vi "Transfer Image Metadata To Host.vi"(0 "image metadata":T1, 1 "reset":bool, 2 "image metadata dma fifo":refnum<k21>, 9 "input valid":bool) -> (4 "overflow":bool, 14 "ready for input":bool)   [LabVIEW 2020, in "GettingStarted_Common_148X_FPGA.lvlib"]
uses:
  GettingStarted_Common_148X_FPGA.lvlib
  Types/Image Metadata.ctl
  <instrlib>/FlexRIO/CSI-2/v2/Common/Types/LLP Data Type.ctl
  <vilib>/rvi/DataTransferAndStorage/Container/Common/niFpgaContainerExecOnDevCompGetState.vi
  <vilib>/rvi/Emulation/niFpgaSctlEmulationGetInTimedLoop.vi
  <vilib>/rvi/errors/niFpgaSetErrorForExecOnDevCompSimple.vi
  <vilib>/rvi/eio/common/nirviEmuReportErrorAndStop.vi
  <vilib>/rvi/interface/RandomDataEmulation/nirviRandomDataAcquireLock.vi
  <vilib>/rvi/interface/RandomDataEmulation/nirviRandomDataQueueStore.vi
  <vilib>/rvi/interface/RandomDataEmulation/nirviRandomDataReleaseLock.vi
  <vilib>/rvi/interface/RandomDataEmulation/nirviFPGAContextMergeError.vi
  <vilib>/rvi/interface/RandomDataEmulation/nirviRandomDataCheckExitLoopConditions.vi
  <vilib>/express/rvi/timingcommon/nirviCommon.vi
  <vilib>/rvi/interface/RandomDataEmulation/niFpgaRandomDataHandleErrors.vi
  <vilib>/rvi/DataTransferAndStorage/Container/XNode/niFpgaContainer.xnode
  <vilib>/rvi/FIFO/Fifo_Resource/niFpgaFifoEmulationRefInMultiElement.vi
  <instrlib>/_niInstr/Basic Elements/v1/FPGA/niInstr Basic Elements v1 FPGA.lvlib
  <instrlib>/FlexRIO/CSI-2/v2/Common/NI CSI-2 API Common v2.lvlib
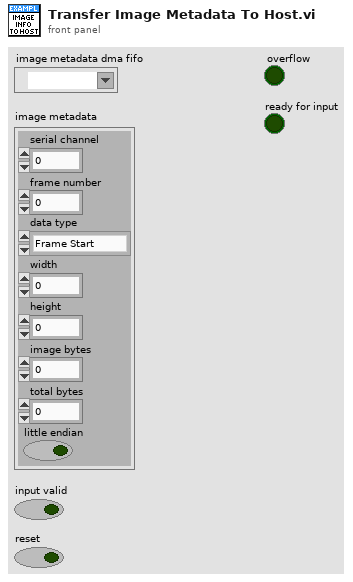
[diagram p1: front panel]
types:
  T1 = typedef "GettingStarted_Common_148X_FPGA.lvlib/Image Metadata.ctl" = cluster{"serial channel":fxp<+,3,3>, "frame number":u16, "data type":T2, "width":u16, "height":u16, "image bytes":u32, "total bytes":u32, "little endian":bool}
  T2 = typedef "NI CSI-2 API Common v2.lvlib/LLP Data Type.ctl" = enum8{"Frame Start", "Frame End", "Line Start", "Line End", "End of Transmission", "Reserved 0", "Reserved 1", "Reserved 2", "Generic Short Packet 1", "Generic Short Packet 2", "Generic Short Packet 3", "Generic Short Packet 4", "Generic Short Packet 5", "Generic Short Packet 6", "Generic Short Packet 7", "Generic Short Packet 8", "Null", "Blanking Data", "Embedded 8-bit non Image Data", "Generic Long Packet 1", "Generic Long Packet 2", "Generic Long Packet 3", "Generic Long Packet 4", "Reserved 3", "YUV420 8-bit", "YUV420 10-bit", "Legacy YUV420 8-bit", "Reserved 4", "YUV420 8-bit Chroma Shifted", "YUV420 10-bit Chroma Shifted", "YUV422 8-bit", "YUV422 10-bit", "RGB444", "RGB555", "RGB565", "RGB666", "RGB888", "Reserved 5", "Reserved 6", "RAW 24", "RAW 6", "RAW 7", "RAW 8", "RAW 10", "RAW 12", "RAW 14", "RAW 16", "RAW 20", "User Defined 8-bit Data 1", "User Defined 8-bit Data 2", "User Defined 8-bit Data 3", "User Defined 8-bit Data 4", "User Defined 8-bit Data 5", "User Defined 8-bit Data 6", "User Defined 8-bit Data 7", "User Defined 8-bit Data 8", "USL Command", "Reserved 7", "Reserved 8", "Reserved 9", "Reserved 10", "Reserved 11", "Reserved 12", "LRTE EPD Spacer"}
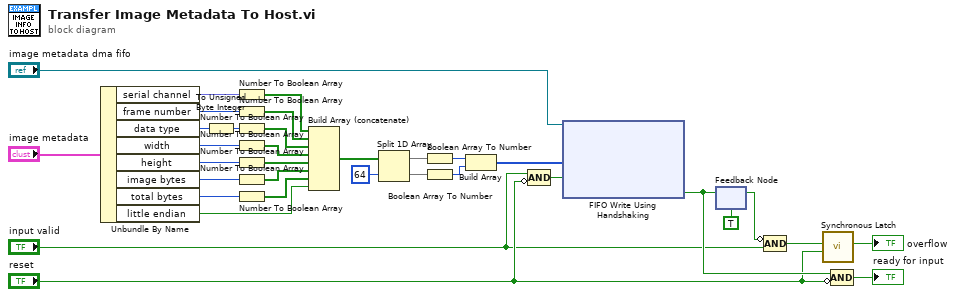
[diagram p0: block diagram]
diagram:
  n1 = Unbundle By Name("image metadata") -> ("serial channel"=w2:fxp<+,3,3>, "frame number"=w32:u16, "data type"=w31:T2, "width"=w30:u16, "height"=w29:u16, "image bytes"=w28:u32, "total bytes"=w21:u32, "little endian"=w4:bool)
  n2 = To Unsigned Byte Integer(number=w31) -> (unsigned 8bit integer=w27:u8)
  n3 = Number To Boolean Array(number=w2) -> (Boolean array=w1:bool[])
  n4 = Number To Boolean Array(number=w32) -> (Boolean array=w26:bool[])
  n5 = Number To Boolean Array(number=w27) -> (Boolean array=w25:bool[])
  n6 = Number To Boolean Array(number=w30) -> (Boolean array=w24:bool[])
  n7 = Number To Boolean Array(number=w29) -> (Boolean array=w23:bool[])
  n8 = Number To Boolean Array(number=w28) -> (Boolean array=w22:bool[])
  n9 = Number To Boolean Array(number=w21) -> (Boolean array=w3:bool[])
  n10 = Build Array (concatenate)(w1, w26, w25, w24, w23, w22, w3, w4) -> (w20:bool[])
  n11 = Split 1D Array(array=w20, index=64) -> (first subarray=w18:bool[], second subarray=w17:bool[])
  n12 = Boolean Array To Number(Boolean array=w18) -> (number=w16:u64)
  n13 = Boolean Array To Number(Boolean array=w17) -> (number=w15:u64)
  n14 = Build Array(w16, w15) -> (w14:u64[])
  n15 = Compound Arithmetic op=AND("input valid", invert "reset") -> (w5:bool)
  n16 = xnode ("FIFO Write Using Handshaking")("Element"=w14, "Input Valid"=w5, "FIFO In"="image metadata dma fifo") -> ("Ready for Input"=w10:bool)  [unwired: 1 out]
  n17 = feedback-in #1(w10) -> ()
  n18 = feedback #1(TRUE ("Ready for Input")) -> (w9:bool)
  n19 = Compound Arithmetic op=AND(invert w9, "input valid") -> (w12:bool)
  n20 = call <instrlib>:"Synchronous Latch.vi"("clear"="reset", "set"=w12) -> ("out"=→"overflow":bool)  [unwired: 9 in]
  n21 = Compound Arithmetic op=AND(w10, invert "reset") -> (→"ready for input":bool)
